vi "AccelerometerGetAcceleration.vi"(0 "error in (no error)":errorcluster, 3 "Device In":u64) -> (7 "error out":errorcluster, 9 "Acceleration":dbl[](array[numeric]), 10 "Device Out":u64)   [LabVIEW 2012, in "Phidget Accelerometer.lvlib"]
doc: "${Acceleration:Header}"
uses:
  <instrlib>/Phidgets/Phidget Accelerometer/Phidget Accelerometer.lvlib
  <instrlib>/Phidgets/Phidget Common/Phidget Common.lvlib
  phidget22.dll
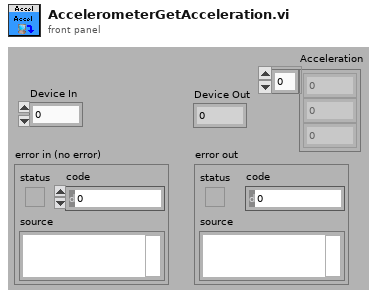
[diagram p1: front panel]
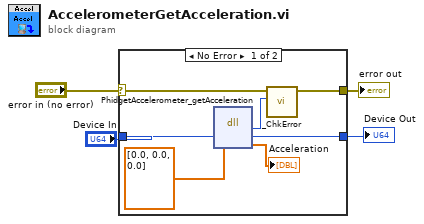
[diagram p0: block diagram]
diagram:
  n1 = case shown="No Error" "error in (no error)" {
    selector: "error in (no error)" -> [w9 w13]
    tunnel: [w8 w13] -> w3
    tunnel: "Device In" -> [w11 w12]
    tunnel: [w10 w12] -> w2
    frame No Error {
      n2 = dll-call lib="phidget22.*" fn="PhidgetAccelerometer_getAcceleration"("phid"=w11, "accelerations"=dbl[] [0.0, 0.0, 0.0]) -> ("return type"=w7:i32, "phid"=w10:u64, "accelerations"=→"Acceleration":dbl[])  [unwired: 3 in, 2 out]
      n3 = call <instrlib>:"_ChkError.vi"("Return Code"=w7, "error in (no error)"=w9) -> ("error out"=w8:errorcluster)  [unwired: 9 in]
    }
    frame Error {
    }
  }
  "error out" <- w3
  "Device Out" <- w2
